vi "Configure Memory and Vacuum.vi"(8 "error in (no error)":errorcluster, 9 "Memory Location (000)":i16 min=0 max=511 step=1 format="%03.0f", 10 "Vacuum Setting (0000)":i64 min=0 max=180 step=1 format="%04.0f", 11 "VISA resource name":refnum<visa-resource-name>) -> (0 "error out":errorcluster, 3 "VISA resource name out":refnum<visa-resource-name>)   [LabVIEW 2016, in "EFD Ultimus V.lvlib"]
doc: "Updates the vacuum value in the memory location specified in the command. This command will update the LCD screen to the specified memory location.\n\nHost Format: VH--CHcccVvvvv\n ccc:The 3 digit memory location from 0-399.\n vvvv:The four digit vacuum setting exlcluding the decimal point. This is a unit less value. The valid \n vacuum ranges and decimal point are determined by the vacuum units currently selected in the \n dispenser."
uses:
  EFD Ultimus V.lvlib
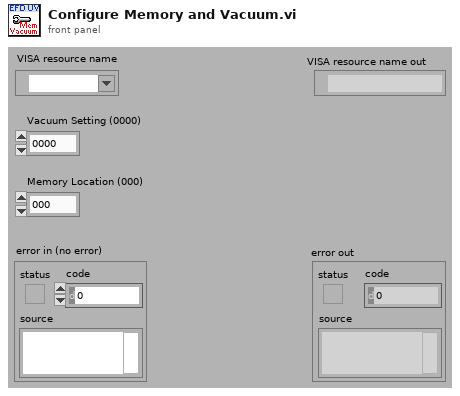
[diagram p1: front panel]
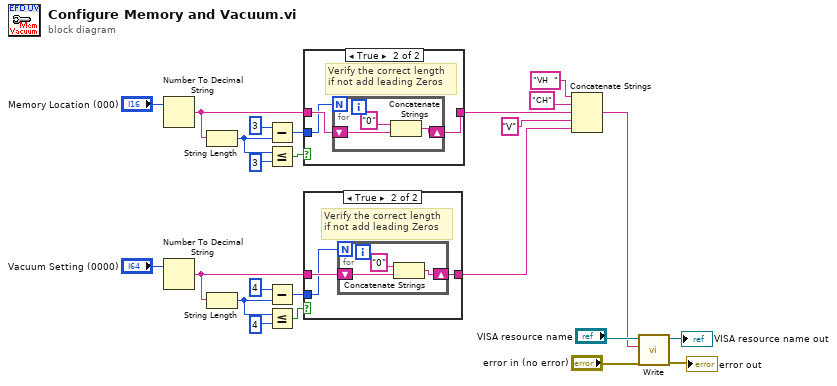
[diagram p0: block diagram]
diagram:
  n1 = Number To Decimal String(number="Memory Location (000)") -> (decimal integer string=w13:string)  [unwired: 1 out]
  n2 = Number To Decimal String(number="Vacuum Setting (0000)") -> (decimal integer string=w23:string)  [unwired: 1 out]
  n3 = String Length(string=w13) -> (length=w15:i32)
  n4 = String Length(string=w23) -> (length=w22:i32)
  n5 = Subtract(x=3, y=w15) -> (x-y=w17:i32)
  n6 = Less Or Equal?(x=w15, y=3) -> (x <= y?=w12:bool)
  n7 = Subtract(x=4, y=w22) -> (x-y=w18:i32)
  n8 = Less Or Equal?(x=w22, y=4) -> (x <= y?=w20:bool)
  n9 = case shown="True" w12 {
    tunnel: w13 -> [w25 w28]
    tunnel: [w25 w27] -> w14
    tunnel: w17 -> [_ w26]
    frame False {
    }
    frame True {
      # "Verify the correct length\nif not add leading Zeros"
      n10 = for {
        N: w26 -> [_]
        shift-right: [w30] -> w27
        shift-left: w28 -> [w29]
        n11 = Concatenate Strings("0" ("string"), w29) -> (w30:string)
      }
    }
  }
  n12 = case shown="True" w20 {
    tunnel: w23 -> [w32 w35]
    tunnel: [w32 w34] -> w24
    tunnel: w18 -> [_ w33]
    frame False {
    }
    frame True {
      # "Verify the correct length\nif not add leading Zeros"
      n13 = for {
        N: w33 -> [_]
        shift-right: [w37] -> w34
        shift-left: w35 -> [w36]
        n14 = Concatenate Strings("0" ("string"), w36) -> (w37:string)
      }
    }
  }
  n15 = Concatenate Strings("VH  " ("string"), "CH" ("string"), w14, "V" ("string"), w24) -> (w3:string)
  n16 = call "Write.vi"("error in (no error)"="error in (no error)", "Command To Write"=w3, "VISA resource name"="VISA resource name") -> ("error out"=→"error out":errorcluster, "VISA resource name out"=→"VISA resource name out":refnum<visa-resource-name>)  [unwired: 7 out]
